vi "GEA2 Script_Parser Core.vi"(0 "Script In":string, 5 "Default wait time (s)":dbl, 7 "Default continue if failed?":bool, 11 "Error In":errorcluster) -> (4 "Script Output":T1[](array[typedef]), 15 "Error Out":errorcluster)   [LabVIEW 2014]
doc: "This VI parses a GEA2 script file and returns a 1D array of test case names and a 2D array of the respective test case commands."
uses:
  typedefs/Script Output.ctl
  typedefs/Command Type.ctl
  typedefs/Command Type String Array.ctl
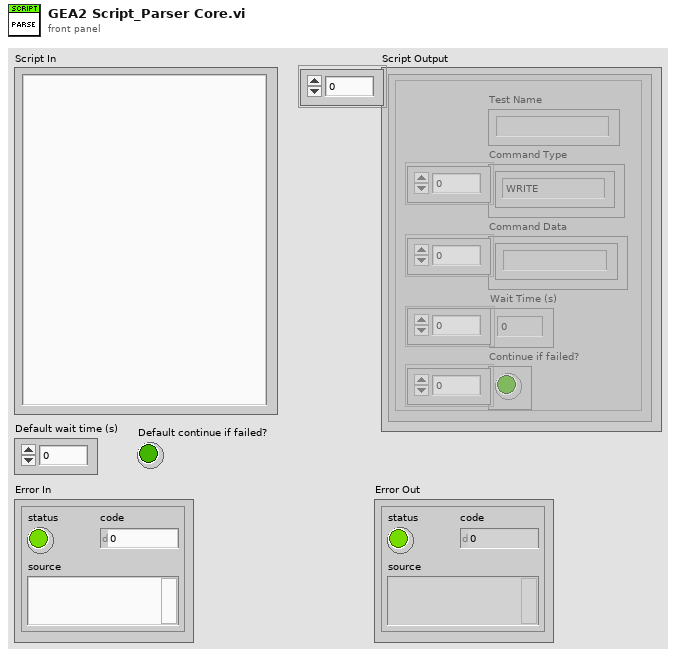
[diagram p1: front panel]
types:
  T1 = typedef "Script Output.ctl" = cluster{"Command Data":string[], "Command Type":T2[], "Test Name":string, "Wait Time (s)":dbl[], "Continue if failed?":bool[]}
  T2 = typedef "Command Type.ctl" = enum16{"WRITE", "READ", "ERDWRITE", "ERDREAD"}
  T3 = typedef "Command Type String Array.ctl" = string[]
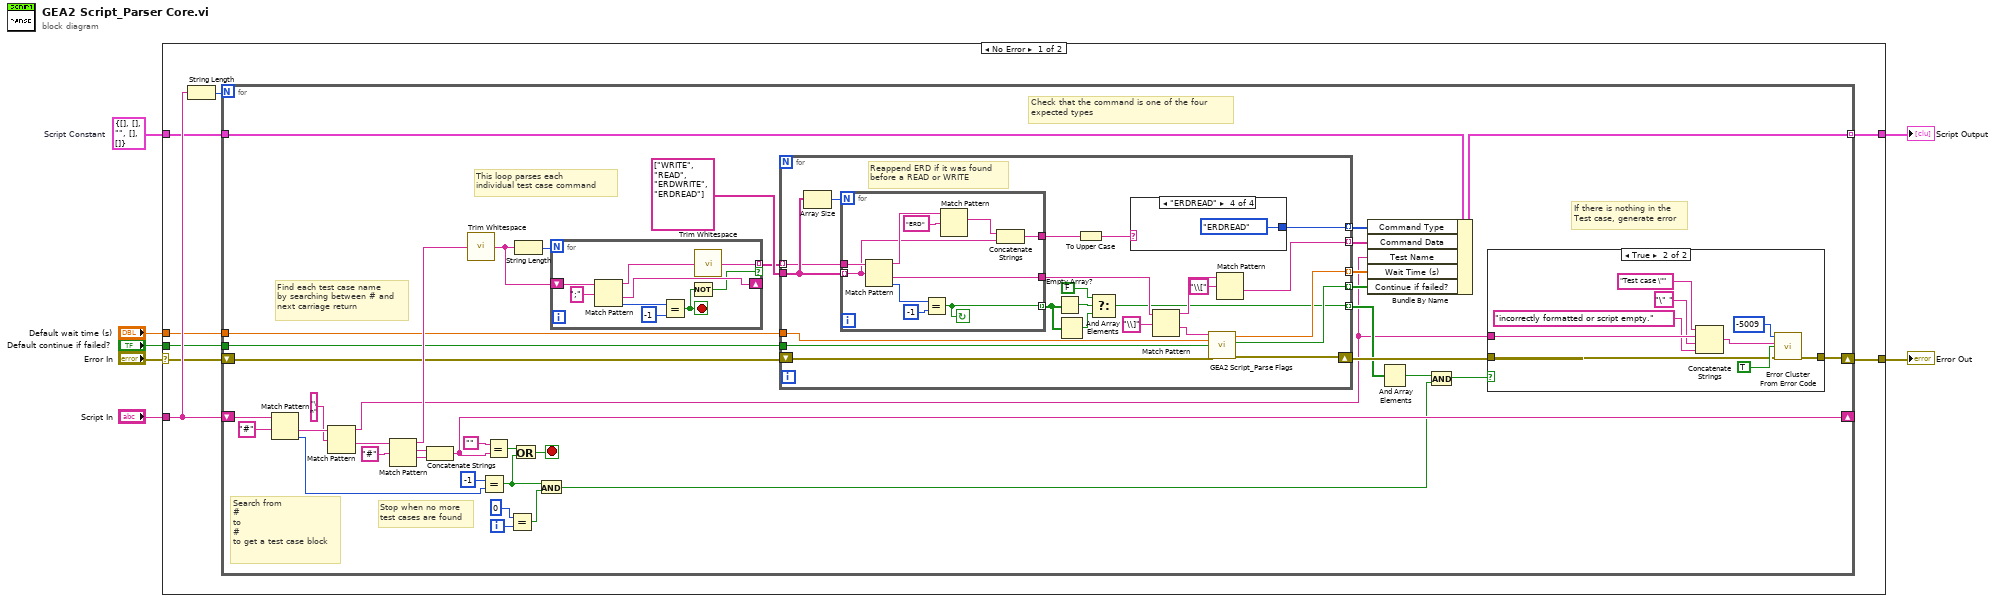
[diagram p0: block diagram]
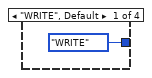
[diagram p2: hidden frame]
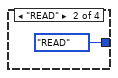
[diagram p3: hidden frame]
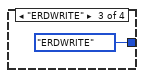
[diagram p4: hidden frame]
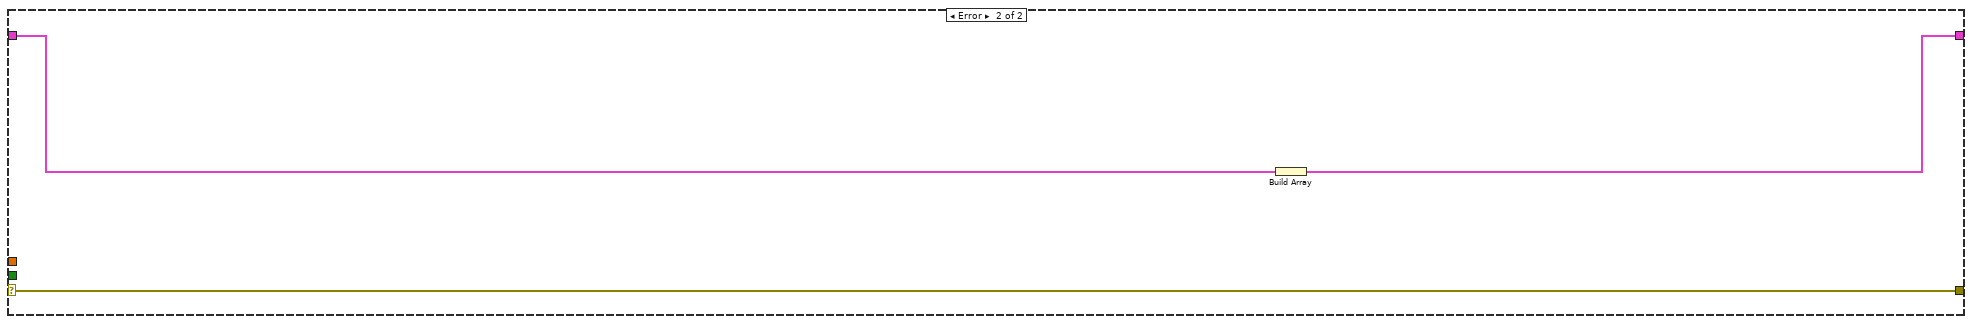
[diagram p6: hidden frame]
diagram:
  w2 = T1 {"Command Data"=[], "Command Type"=[], "Test Name"="", "Wait Time (s)"=[], "Continue if failed?"=[]}  # Script Constant
  n1 = case shown="No Error" "Error In" {
    selector: "Error In" -> [w12 w113]
    tunnel: "Script In" -> [w14 _]
    tunnel: [w13 w113] -> w5
    tunnel: "Default continue if failed?" -> [w11 _]
    tunnel: "Default wait time (s)" -> [w10 _]
    tunnel: w2 -> [w9 w112]
    tunnel: [w8 w111] -> w1
    frame No Error {
      n2 = String Length(string=w14) -> (length=w15:i32)
      n3 = for {
        N: w15 -> [_]
        shift-right: [w28] -> _
        shift-left: w14 -> [w51]
        shift-right: [w37] -> w13
        shift-left: w12 -> [w32]
        tunnel: w11 -> [w35]
        tunnel: w10 -> [w34]
        tunnel: w9 -> [w24]
        tunnel: [w25] -> w8 mode=indexing
        i -> [w21]
        stop <- w44 stop-if-true
        # "Find each test case name\nby searching between # and\nnext carriage return"
        # "This loop parses each\nindividual test case command"
        # "Check that the command is one of the four\nexpected types"
        # "If there is nothing in the\nTest case, generate error"
        # "Stop when no more\ntest cases are found"
        # "Search from\n#\nto\n#\nto get a test case block"
        n4 = Match Pattern(string=w51, regular expression="#") -> (after substring=w41:string, offset past match=w53:i32)  [unwired: 1 in, 2 out]
        n5 = Match Pattern(string=w41, regular expression="\n") -> (before substring=w27:string, after substring=w39:string)  [unwired: 1 in, 2 out]
        n6 = Match Pattern(string=w39, regular expression="#") -> (before substring=w45:string, match substring=w50:string, after substring=w49:string)  [unwired: 1 in, 1 out]
        n7 = Concatenate Strings(w50, w49) -> (w28:string)
        n8 = call <vilib>:"Trim Whitespace.vi"("string"=w45) -> ("trimmed string"=w42:string)  [unwired: 1 in]
        n9 = Equal?(x=-1, y=w53) -> (x = y?=w23:bool)
        n10 = Equal?(x="", y=w28) -> (x = y?=w47:bool)
        n11 = Equal?(x=0, y=w21) -> (x = y?=w22:bool)
        n12 = Or(x=w47, y=w23) -> (x .or. y?=w44:bool)
        n13 = String Length(string=w42) -> (length=w43:i32)
        n14 = And(x=w23, y=w22) -> (x .and. y?=w17:bool)
        n15 = for {
          N: w43 -> [_]
          shift-right: [w104] -> _
          shift-left: w42 -> [w108]
          tunnel: [w106] -> w36 mode=indexing if=w102
          stop <- w103 stop-if-true
          n16 = Match Pattern(string=w108, regular expression=";") -> (before substring=w107:string, after substring=w104:string, offset past match=w109:i32)  [unwired: 1 in, 1 out]
          n17 = Equal?(x=w109, y=-1) -> (x = y?=w103:bool)
          n18 = Not(x=w103) -> (.not. x?=w102:bool)
          n19 = call <vilib>:"Trim Whitespace.vi"("string"=w107) -> ("trimmed string"=w106:string)  [unwired: 1 in]
        }
        n20 = for {
          tunnel: w36 -> [w57] mode=indexing
          tunnel: T3 ["WRITE", "READ", "ERDWRITE", "ERDREAD"] -> [w76]
          tunnel: [w63] -> w26 mode=indexing
          tunnel: w35 -> [w72]
          tunnel: w34 -> [w71]
          shift-right: [w70] -> w33
          shift-left: w32 -> [w69]
          tunnel: [w58] -> w31 mode=indexing
          tunnel: [w68] -> w30 mode=indexing
          tunnel: [w67] -> w29 mode=indexing
          tunnel: [w66] -> w16 mode=indexing
          # "Reappend ERD if it was found\nbefore a READ or WRITE"
          n21 = Array Size(array=w76) -> (size(s)=w77:i32)
          n22 = for {
            N: w77 -> [_]
            tunnel: w76 -> [w85] mode=indexing
            tunnel: [w84] -> w55
            tunnel: w57 -> [w89]
            tunnel: [w83] -> w75
            tunnel: [w82] -> w62 mode=indexing
            stop <- w82 continue-if-true
            n23 = Match Pattern(string=w89, regular expression=w85) -> (before substring=w88:string, after substring=w83:string, offset past match=w91:i32)  [unwired: 1 in, 1 out]
            n24 = Equal?(x=w91, y=-1) -> (x = y?=w82:bool)
            n25 = Match Pattern(string=w88, regular expression="ERD") -> (match substring=w86:string)  [unwired: 1 in, 3 out]
            n26 = Concatenate Strings(w86, w85) -> (w84:string)
          }
          n27 = Empty Array?(array=w62) -> (empty?=w61:bool)
          n28 = And Array Elements(Boolean array=w62) -> (logical AND=w59:bool)
          n29 = To Upper Case(1:w55) -> (0:w56:string)
          n30 = Select(t=FALSE, s=w61, f=w59) -> (s? t:f=w58:bool)
          n31 = case shown="\"ERDREAD\"" w56 {
            tunnel: [Command_Type."WRITE" ("Command Type") Command_Type."READ" ("Command Type") Command_Type."ERDWRITE" ("Command Type") Command_Type."ERDREAD" ("Command Type")] -> w66
            frame "WRITE", Default {
            }
            frame "READ" {
            }
            frame "ERDWRITE" {
            }
            frame "ERDREAD" {
            }
          }
          n32 = Match Pattern(string=w75, regular expression="\\]") -> (before substring=w65:string, after substring=w73:string)  [unwired: 1 in, 2 out]
          n33 = call "GEA2 Script_Parse Flags.vi"("Flag String"=w73, "Default wait time (s)"=w71, "Default Continue if stopped?"=w72, "Error In"=w69) -> ("Wait time (s)"=w67:dbl, "Continue if stopped?"=w68:bool, "Error Out"=w70:errorcluster)  [unwired: 9 in]
          n34 = Match Pattern(string=w65, regular expression="\\[") -> (after substring=w63:string)  [unwired: 1 in, 3 out]
        }
        n35 = Bundle By Name(cluster=w24, "Command Type"=w16, "Command Data"=w26, "Test Name"=w27, "Wait Time (s)"=w29, "Continue if failed?"=w30) -> (w25:T1)
        n36 = And Array Elements(Boolean array=w31) -> (logical AND=w18:bool)
        n37 = And(x=w18, y=w17) -> (x .and. y?=w19:bool)
        n38 = case shown="True" w19 {
          tunnel: w33 -> [w92 w96]
          tunnel: [w92 w95] -> w37
          tunnel: w27 -> [_ w100]
          frame False {
          }
          frame True {
            n39 = Concatenate Strings("Test case \"" ("string"), w100, "\" " ("string"), "incorrectly formatted or script empty." ("string")) -> (w93:string)
            n40 = call <vilib>:"Error Cluster From Error Code.vi"("show call chain? (False)"=TRUE, "error in (no error)"=w96, "error message (\"\")"=w93, "error code (0)"=-5009 ("code")) -> ("error out"=w95:errorcluster)  [unwired: 5 in]
          }
        }
      }
    }
    frame Error {
      n41 = Build Array(w112) -> (w111:T1[])
    }
  }
  "Error Out" <- w5
  "Script Output" <- w1
